vi "subVI_Strain.vi"(4 "timeout (s)":dbl=10.0 caption="타임아웃(초)" format="%0.2f", 5 "error in":errorcluster caption="에러 입력", 7 "stop (T)":bool=TRUE caption="정지(T)", 10 "디바이스 이름":tag="cDAQ1Mod7") -> (14 "task out":refnum<k21> caption="태스크 출력", 15 "data":bool[](array[boolean]) caption="데이터", 19 "error out":errorcluster caption="에러 출력")   [LabVIEW 2013]
doc: "NI-DAQmx를 사용하여 태스크를 생성, 편집, 실행합니다. NI-DAQmx가 지원하는 디바이스의 완전한 리스트는 NI-DAQ Readme를 참조하십시오.\n\n이 익스프레스 VI를 블록다이어그램에 놓으면 DAQ 어시스턴트가 시작되어 새로운 태스크를 생성합니다, 태스크를 생성한 후, DAQ 어시스턴트 익스프레스 VI를 더블 클릭하여 해당 태스크를 편집할 수 있습니다. 연속적인 측정 또는 생성을 위해서는 DAQ 어시스턴트 익스프레스 주위에 while 루프를 놓습니다.\n\n연속적인 단일 포인트 입력 또는 출력의 경우 DAQ 어시스턴트 익스프레스 VI는 최적의 성능을 제공하지 않을 수도 있습니다. 높은 성능을 가진 단일 포인트 I/O 어플리케이션을 생성하는 기술에 대한 예제는 examples\\DAQmx\\Analog In\\Measure Voltage.llb의 Cont Acq&Graph Voltage-Single Point Optimization VI를 참조하십시오."
uses:
  <vilib>/DAQmx/read.llb/DAQmx Read.vi
  <vilib>/DAQmx/read.llb/DAQmx Read (Digital 1D Bool NChan 1Samp 1Line).vi
  <vilib>/DAQmx/create/channels.llb/DAQmx Create Channel (DI-Digital Input).vi
  <vilib>/DAQmx/miscellaneous.llb/DAQmx Fill In Error Info.vi
  <resource>/objmgr/daqmx.rc
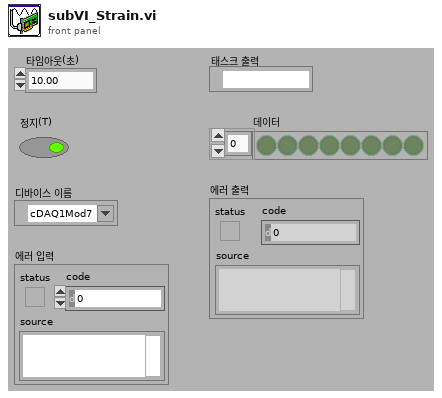
[diagram p1: front panel]
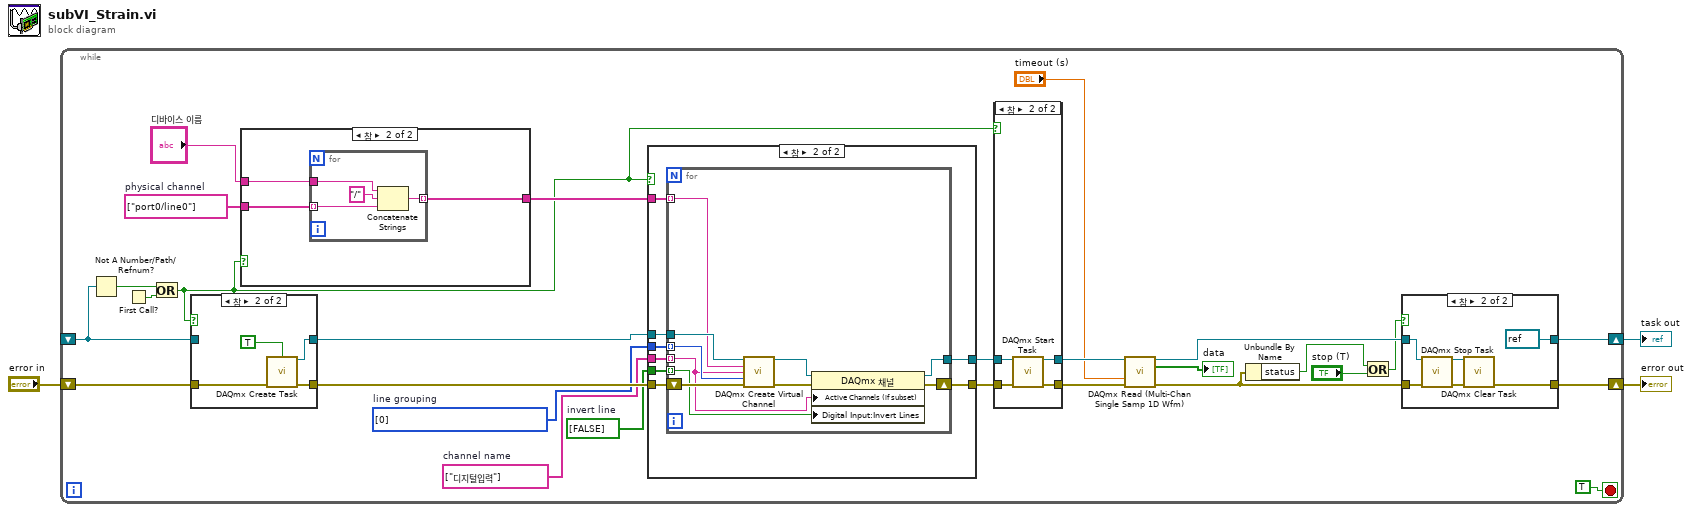
[diagram p0: block diagram]
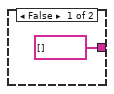
[diagram p5: hidden frame]
diagram:
  n1 = while {
    shift-right: [w10] -> w1
    shift-left: _ -> [w27]
    shift-right: [w8] -> w2
    shift-left: "error in" -> [w28]
    stop <- TRUE stop-if-true
    w18 = bool[] [FALSE]  # invert line
    w19 = i32[] [0] items=["one channel for each line", "one channel for all lines"]  # line grouping
    w20 = string[] ["디지털입력"]  # channel name
    w24 = string[] ["port0/line0"]  # physical channel
    n2 = Not A Number/Path/Refnum?(number/path/refnum=w27) -> (NaN/Path/Refnum?=w26:bool)
    n3 = First Call?() -> (First Call?: T/F=w29:bool)
    n4 = Or(x=w26, y=w29) -> (x .or. y?=w17:bool)
    n5 = case "케이스 구조" shown="참" w17 {
      tunnel: [w74 w78] -> w23
      tunnel: w27 -> [w74 _]
      tunnel: [w73 w77] -> w22
      tunnel: w28 -> [w73 w75]
      frame False {
      }
      frame True {
        n6 = call <vilib>:"DAQmx Create Task.vi"("auto cleanup"=TRUE, "error in"=w75) -> ("task out"=w78:refnum<k21>, "error out"=w77:errorcluster)  [unwired: 12 in]
      }
    }
    n7 = case "케이스 구조" shown="참" w17 {
      tunnel: [string[] [] w68] -> w21
      tunnel: "디바이스 이름" -> [_ w67]
      tunnel: w24 -> [_ w66]
      frame False {
      }
      frame True {
        n8 = for "For 루프" {
          tunnel: [w72] -> w68 mode=indexing
          tunnel: w67 -> [w71]
          tunnel: w66 -> [w69] mode=indexing
          n9 = Concatenate Strings(w71, "/" ("string"), w69) -> (w72:string)
        }
      }
    }
    n10 = case "케이스 구조" shown="참" w17 {
      tunnel: [w46 w47] -> w16
      tunnel: w23 -> [w46 w54]
      tunnel: [w45 w52] -> w15
      tunnel: w22 -> [w45 w53]
      tunnel: w21 -> [_ w51]
      tunnel: w20 -> [_ w50]
      tunnel: w19 -> [_ w49]
      tunnel: w18 -> [_ w48]
      frame False {
      }
      frame True {
        n11 = for "For 루프" {
          tunnel: w54 -> [w62]
          tunnel: w51 -> [w59] mode=indexing
          tunnel: w50 -> [w57] mode=indexing
          tunnel: w49 -> [w58] mode=indexing
          tunnel: w48 -> [w56] mode=indexing
          shift-right: [w60] -> w52
          shift-left: w53 -> [w61]
          tunnel: [w55] -> w47
          n12 = call-poly <vilib>:"DAQmx Create Virtual Channel.vi"("task in"=w62, "lines"=w59, "name to assign"=w57, "line grouping"=w58, "error in"=w61) -> ("task out"=w63:refnum<k21>, "error out"=w64:errorcluster)  [unwired: 9 in]
          n13 = property class="DAQmx 채널"(reference=w63, error in=w64, "Active Channels (if subset)"=w57, "Digital Input:Invert Lines"=w56) -> (reference out=w55:refnum<k21>, error out=w60:errorcluster)
        }
      }
    }
    n14 = case "케이스 구조" shown="참" w17 {
      tunnel: [w40 w43] -> w14
      tunnel: w16 -> [w40 w44]
      tunnel: [w39 w41] -> w13
      tunnel: w15 -> [w39 w42]
      frame False {
      }
      frame True {
        n15 = call <vilib>:"DAQmx Start Task.vi"("task/channels in"=w44, "error in"=w42) -> ("task out"=w43:refnum<k21>, "error out"=w41:errorcluster)  [unwired: 12 in]
      }
    }
    n16 = call-poly "DAQmx Read (Multi-Chan Single Samp 1D Wfm).vi"("task/channels in"=w14, "timeout"="timeout (s)", "error in"=w13) -> ("task out"=w9:refnum<k21>, "data"=→"data":bool[], "error out"=w7:errorcluster)  [unwired: 10 in]
    n17 = Unbundle By Name(w7) -> ("status"=w6:bool)
    n18 = Or(x=w6, y="stop (T)") -> (x .or. y?=w4:bool)
    n19 = case "케이스 구조" shown="참" w4 {
      tunnel: [w32 refnum<k21> refnum ("task in")] -> w10
      tunnel: w9 -> [w32 w38]
      tunnel: [w31 w35] -> w8
      tunnel: w7 -> [w31 w37]
      frame False {
      }
      frame True {
        n20 = call <vilib>:"DAQmx Stop Task.vi"("task/channels in"=w38, "error in"=w37) -> ("task out"=w34:refnum<k21>, "error out"=w36:errorcluster)  [unwired: 12 in]
        n21 = call <vilib>:"DAQmx Clear Task.vi"("task in"=w34, "error in"=w36) -> ("error out"=w35:errorcluster)  [unwired: 13 in]
      }
    }
  }
  "error out" <- w2
  "task out" <- w1
